vi "Configure Acquisition.vi"(8 "error in (no error)":errorcluster, 11 "PWM CFG in":refnum<class "PWM CFG.lvclass">) -> (0 "error out":errorcluster, 3 "PWM CFG out":refnum<class "PWM CFG.lvclass">)   [LabVIEW 2023, in "DIO Simulated.lvlib" / "PWM CFG.lvclass"]
uses:
  PWM CFG.lvclass
  PWM CFG.lvclass/PWM CFG.ctl
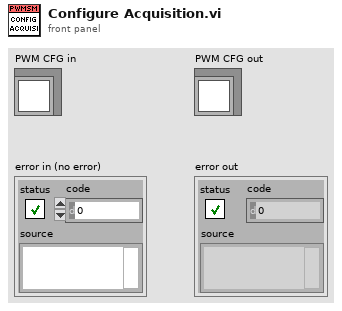
[diagram p1: front panel]
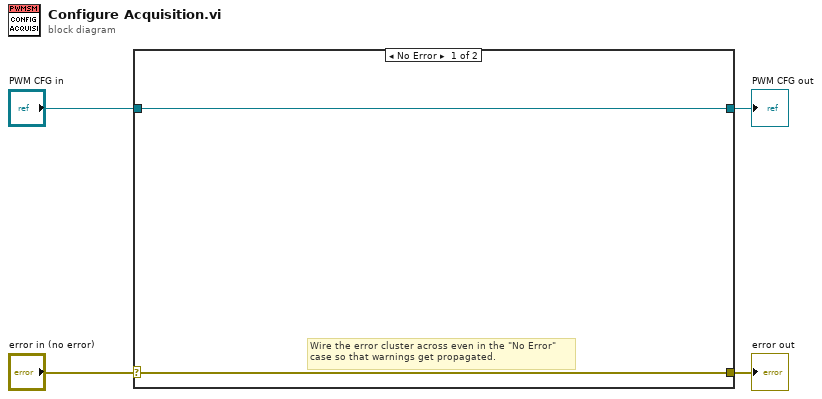
[diagram p0: block diagram]
diagram:
  n1 = case shown="No Error" "error in (no error)" {
    selector: "error in (no error)" -> [w5 w8]
    tunnel: [w5 w8] -> w3
    tunnel: [w6 w7] -> w1
    tunnel: "PWM CFG in" -> [w6 w7]
    frame No Error {
      # "Wire the error cluster across even in the \"No Error\"\ncase so that warnings get propagated."
    }
    frame Error {
    }
  }
  "error out" <- w3
  "PWM CFG out" <- w1
